vi "Write NowTime.vi"(8 "error in (no error)":errorcluster, 10 "NowTime":timestamp, 11 "RealWorkActor in":refnum<class "RealWorkActor.lvclass">) -> (0 "error out":errorcluster, 3 "RealWorkActor out":refnum<class "RealWorkActor.lvclass">)   [LabVIEW 2014, in "RealWorkActor.lvlib" / "RealWorkActor.lvclass"]
uses:
  RealWorkActor.lvclass
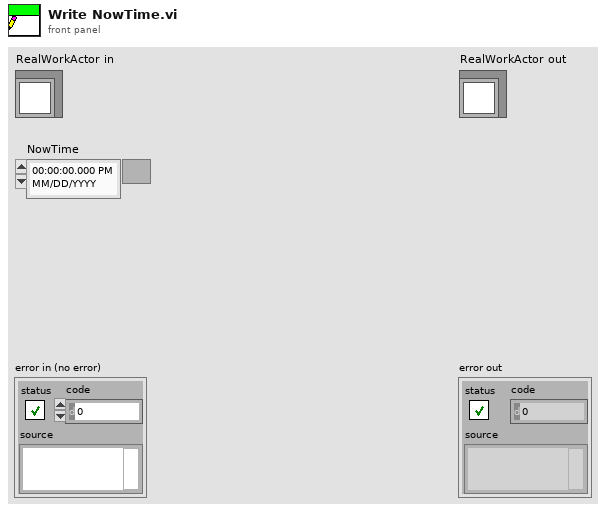
[diagram p1: front panel]
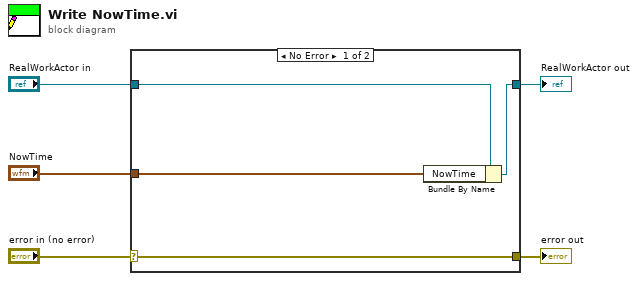
[diagram p0: block diagram]
diagram:
  n1 = case shown="No Error" "error in (no error)" {
    selector: "error in (no error)" -> [w9 w10]
    tunnel: [w9 w10] -> w4
    tunnel: [w7 w11] -> w2
    tunnel: "RealWorkActor in" -> [w8 w11]
    tunnel: "NowTime" -> [w6 _]
    frame No Error {
      n2 = Bundle By Name(cluster=w8, "NowTime"=w6) -> (w7:refnum<class "RealWorkActor.lvclass">)
    }
    frame Error {
    }
  }
  "error out" <- w4
  "RealWorkActor out" <- w2
